vi "run.vi"(8 "error in (no error)":errorcluster, 11 "WasRun in":refnum<class "WasRun.lvclass">) -> (0 "error out":errorcluster, 3 "WasRun out":refnum<class "WasRun.lvclass">)   [LabVIEW 2013, in "WasRun.lvclass"]
uses:
  WasRun.lvclass
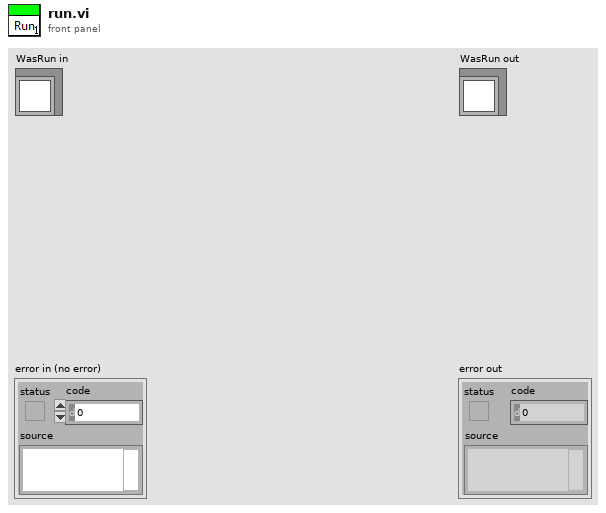
[diagram p1: front panel]
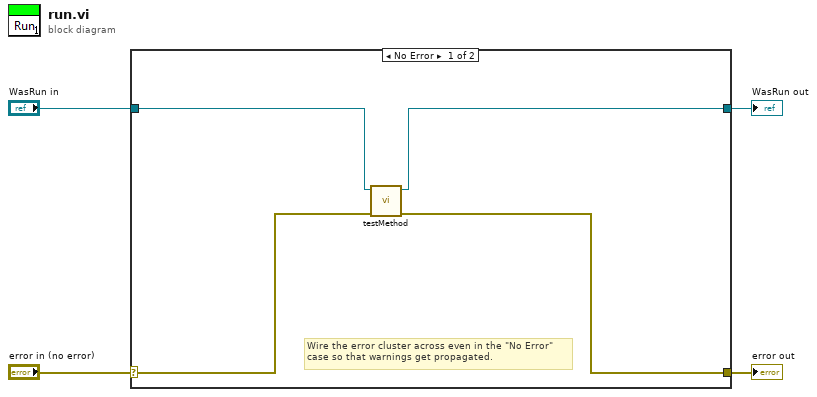
[diagram p0: block diagram]
diagram:
  n1 = case shown="No Error" "error in (no error)" {
    selector: "error in (no error)" -> [w8 w10]
    tunnel: [w5 w10] -> w3
    tunnel: [w6 w9] -> w1
    tunnel: "WasRun in" -> [w7 w9]
    frame No Error {
      # "Wire the error cluster across even in the \"No Error\"\ncase so that warnings get propagated."
      n2 = call-dynamic "testMethod.vi"("error in (no error)"=w8, "WasRun in"=w7) -> ("error out"=w5:errorcluster, "WasRun out"=w6:refnum<class "WasRun.lvclass">)  [unwired: 8 in]
    }
    frame Error {
    }
  }
  "error out" <- w3
  "WasRun out" <- w1
